vi "zStackIncreasePowerGUI.vi"() -> ()   [LabVIEW 2011]
panel:
  in  "Motor":string(combo)="stage.z"
  in  "Cluster":T1={"Start-power"=0.02, "double distance"=0.0001} {"double distance" min=0.0 max=0.00025 step=1e-06 format="%#_6p"; "Start-power" format="%#_3p"}
  in  "cancel":bool
  in  "Get end":bool
  in  "Get start":bool
  in  "job name":string="z-Stack"
  in  "close":bool
  out "Slices":u16=100
  in  "distance":dbl=1.0000000000000002e-06 min=0.0 max=0.00025 step=1e-07 format="%#_6p"
  in  "Start":bool
  in  "end":dbl=0.00015 min=1e-06 max=0.02 step=1e-06 format="%#_6p"
  in  "start":dbl=5e-05 min=0.0 max=0.02 step=1e-06 format="%#_6p"
  # "daten,i vom Globaldata holen, im globaldata i+1,"
  # "use u for µm"
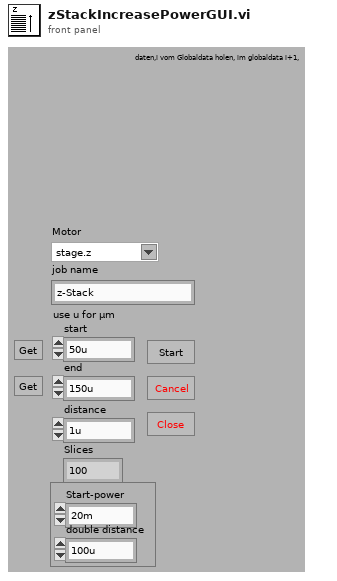
[diagram p1: front panel]
types:
  T1 = cluster{"Start-power":dbl, "double distance":dbl}
  T2 = enum16{"None/#Datasets", "Clear", "TagValueOf#", "AddValues", "ReadValue", "ChangeValue", "Get all"}
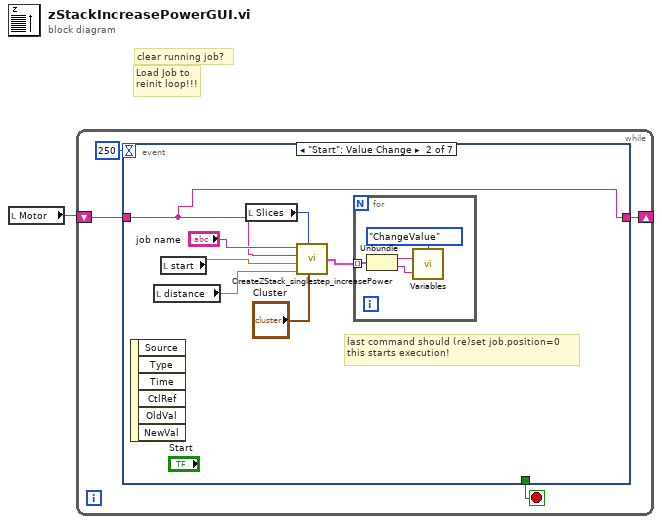
[diagram p0: block diagram]
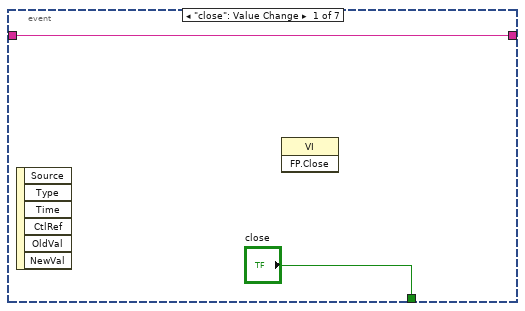
[diagram p2: hidden frame]
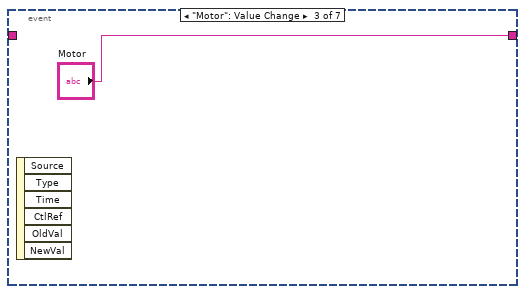
[diagram p3: hidden frame]
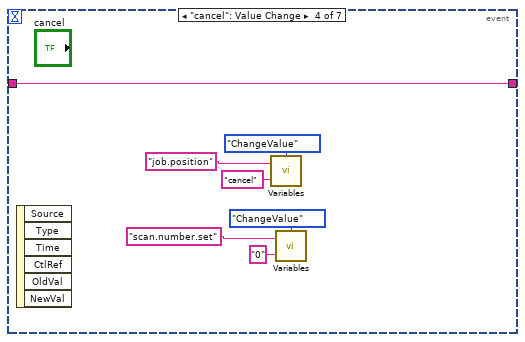
[diagram p4: hidden frame]
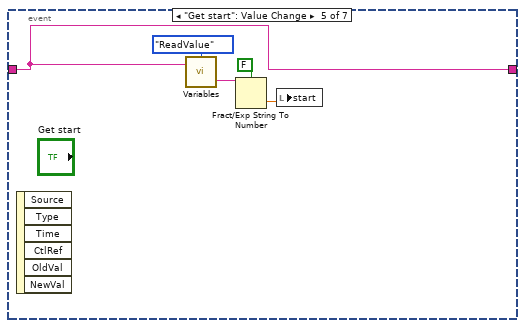
[diagram p5: hidden frame]
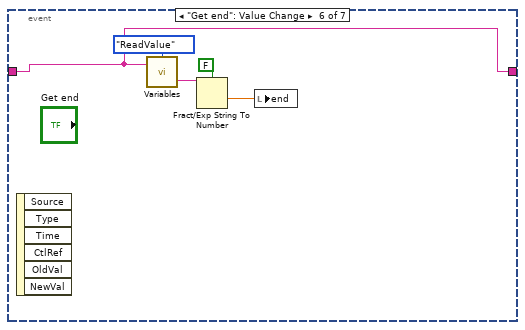
[diagram p6: hidden frame]
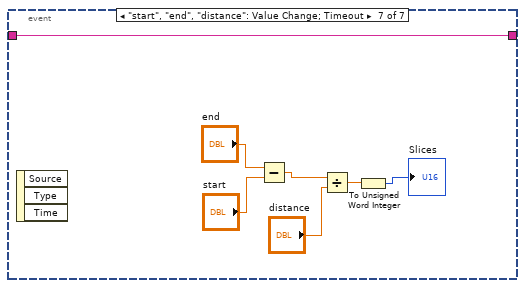
[diagram p7: hidden frame]
diagram:
  # "Load Job to\nreinit loop!!!"
  # "clear running job?"
  n1 = local read "Motor"() -> (w1:string)
  n2 = while {
    shift-right: [w3] -> _
    shift-left: w1 -> [w2]
    stop <- w5 stop-if-true
    n3 = event shown="[1] \"Start\": Value Change" {
      selector: _ -> [_ _ _ _ _ _ _]
      dyn-events: _ -> [_ _ _ _ _ _ _]
      timeout: 250 -> [_ _ _ _ _ _ _]
      tunnel: ["close" _ _ _ _ _ _] -> w5
      tunnel: [w6 w8 "Motor" w20 w27 w32 w37] -> w3
      tunnel: w2 -> [w6 w8 _ w20 w27 w32 w37]
      event "close": Value Change {
        n4 = event-data() -> ()  [unwired: 7 out]
        n5 = invoke class="VI" method="FP.Close"() -> ()  [unwired: 3 in, 3 out]
      }
      event "Start": Value Change {
        # "last command should (re)set job.position=0\nthis starts execution!"
        n6 = event-data() -> ()  [unwired: 7 out]
        n7 = local read "distance"() -> (w12:dbl)
        n8 = local read "start"() -> (w13:dbl)
        n9 = local read "Slices"() -> (w11:u16)
        n10 = call "CreateZStack_singlestep_increasePower.vi"("Cluster"="Cluster", "Slices"=w11, "distance"=w12, "start"=w13, "motor"=w8, "job name"="job name") -> ("Z-Stack array"=w10:cluster{string, "job name":string}[])
        n11 = for {
          tunnel: w10 -> [w17] mode=indexing
          n12 = Unbundle(w17) -> (w16:string, "job name"=w15:string)
          n13 = call "Variables.vi"("value"=w15, "Tag in"=w16, "Command"=T2."ChangeValue") -> ()  [unwired: 3 out]
        }
      }
      event "Motor": Value Change {
        n14 = event-data() -> ()  [unwired: 7 out]
      }
      event "cancel": Value Change {
        n15 = event-data() -> ()  [unwired: 7 out]
        n16 = call "Variables.vi"("value"="cancel", "Tag in"="job.position" ("name (unnamed)"), "Command"=T2."ChangeValue") -> ()  [unwired: 3 out]
        n17 = call "Variables.vi"("value"="0", "Tag in"="scan.number.set" ("name (unnamed)"), "Command"=T2."ChangeValue") -> ()  [unwired: 3 out]
      }
      event "Get start": Value Change {
        n18 = event-data() -> ()  [unwired: 7 out]
        n19 = call "Variables.vi"("Tag in"=w27, "Command"=T2."ReadValue") -> ("value out"=w30:string)  [unwired: 1 in, 2 out]
        n20 = Fract/Exp String To Number(use system decimal point (T)=FALSE, string=w30) -> (number=w28:dbl)  [unwired: 3 out]
        n21 = local write "start"(w28) -> ()
      }
      event "Get end": Value Change {
        n22 = event-data() -> ()  [unwired: 7 out]
        n23 = call "Variables.vi"("Tag in"=w32, "Command"=T2."ReadValue") -> ("value out"=w35:string)  [unwired: 1 in, 2 out]
        n24 = Fract/Exp String To Number(use system decimal point (T)=FALSE, string=w35) -> (number=w33:dbl)  [unwired: 3 out]
        n25 = local write "end"(w33) -> ()
      }
      event "start", "end", "distance": Value Change; Timeout {
        n26 = event-data() -> ()  [unwired: 4 out]
        n27 = Subtract(x="end", y="start") -> (x-y=w41:dbl)
        n28 = Divide(x=w41, y="distance") -> (x/y=w39:dbl)
        n29 = To Unsigned Word Integer(number=w39) -> (unsigned 16bit integer=→"Slices":u16)
      }
    }
  }
